vi "GetAllVariables.vi"(10 "Ftp":refnum<k24>, 11 "error in":errorcluster) -> (2 "Variable files":T1(array[cluster]), 3 "error out":errorcluster)   [LabVIEW 2010, in "UnderAutomation.Fanuc.lvlib"]
uses:
  UnderAutomation.Fanuc.lvlib
  C:/Users/fg/Documents/Fanuc.vi/LabVIEW_2024/UnderAutomation.Fanuc/lib/UnderAutomation.Fanuc.dll
  LabVIEW_2024/UnderAutomation.Fanuc/lib/UnderAutomation.Fanuc.dll
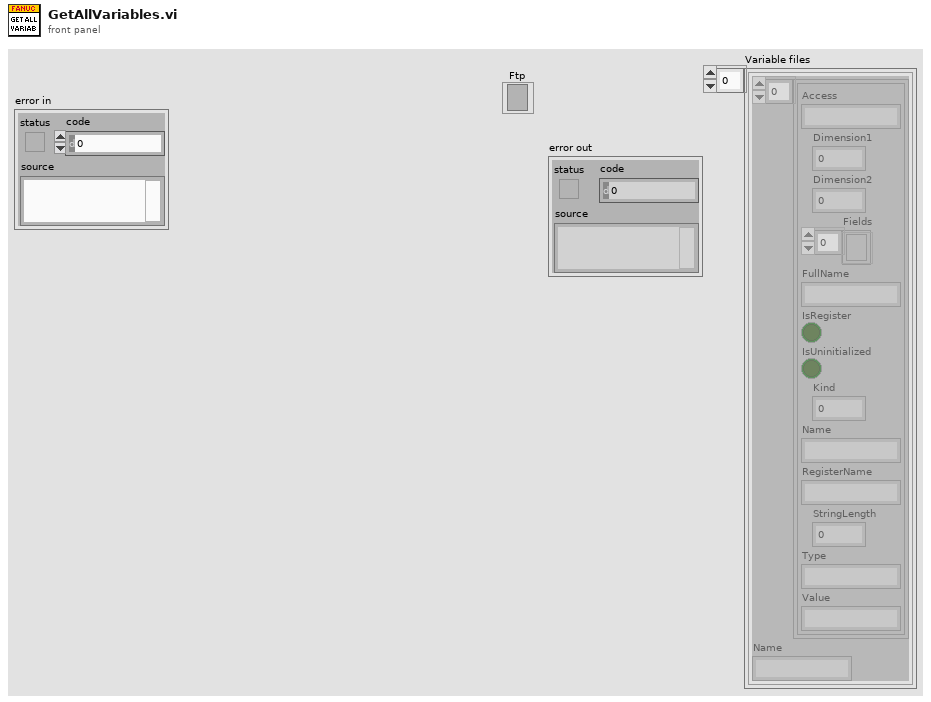
[diagram p1: front panel]
types:
  T1 = cluster{cluster{"Access":string, "Dimension1":i32, "Dimension2":i32, "Fields":refnum<k24>[], "FullName":string, "IsRegister":bool, "IsUninitialized":bool, "Kind":i32, "Name":string, "RegisterName":string, "StringLength":i32, "Type":string, "Value":string}[], "Name":string}[]
  T2 = cluster{"Access":string, "Dimension1":i32, "Dimension2":i32, "Fields":refnum<k24>[], "FullName":string, "IsRegister":bool, "IsUninitialized":bool, "Kind":i32, "Name":string, "RegisterName":string, "StringLength":i32, "Type":string, "Value":string}
  T3 = cluster{cluster{"Access":string, "Dimension1":i32, "Dimension2":i32, "Fields":refnum<k24>[], "FullName":string, "IsRegister":bool, "IsUninitialized":bool, "Kind":i32, "Name":string, "RegisterName":string, "StringLength":i32, "Type":string, "Value":string}[], "Name":string}
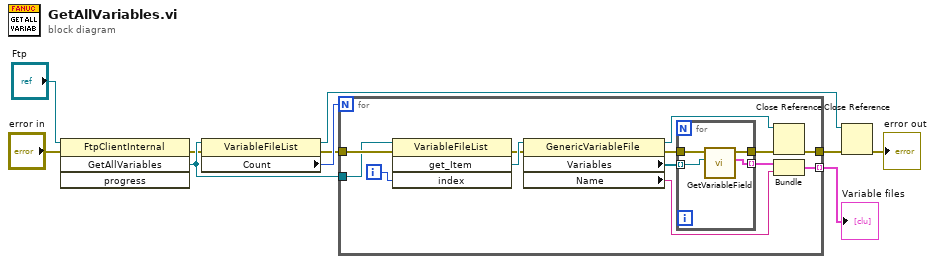
[diagram p0: block diagram]
diagram:
  n1 = invoke class="FtpClientInternal" method="GetAllVariables"(reference="Ftp", error in="error in") -> (error out=w6:errorcluster, "GetAllVariables"=w7:refnum<k24>)  [unwired: 2 in, 2 out]
  n2 = property class="VariableFileList"(reference=w7, error in=w6) -> (reference out=w3:refnum<k24>, error out=w5:errorcluster, "Count"=w8:i32)
  n3 = for {
    N: w8 -> [_]
    tunnel: w7 -> [w22]
    tunnel: w5 -> [w23]
    tunnel: [w15] -> w4 mode=indexing
    tunnel: [w11] -> w2
    i -> [w21]
    n4 = invoke class="VariableFileList" method="get_Item"(reference=w22, error in=w23, "index"=w21) -> (error out=w19:errorcluster, "get_Item"=w20:refnum<k24>)  [unwired: 1 in, 2 out]
    n5 = property class="GenericVariableFile"(reference=w20, error in=w19) -> (reference out=w13:refnum<k24>, error out=w14:errorcluster, "Variables"=w18:refnum<k24>[], "Name"=w16:string)
    n6 = for {
      tunnel: w18 -> [w27] mode=indexing
      tunnel: [w26] -> w17 mode=indexing
      tunnel: [w25] -> w12
      tunnel: w14 -> [w24]
      n7 = call "GetVariableField.vi"("Field"=w27, "error in (no error)"=w24) -> ("Field cluster"=w26:T2, "error out"=w25:errorcluster)  [unwired: 8 in]
    }
    n8 = Close Reference(reference=w13, error in (no error)=w12) -> (error out=w11:errorcluster)
    n9 = Bundle(w17, "Name"=w16) -> (w15:T3)  [unwired: 1 in]
  }
  "Variable files" <- w4
  n10 = Close Reference(reference=w3, error in (no error)=w2) -> (error out=→"error out":errorcluster)
